vi "RemoveConnectionID.vi"(8 "ArrayIN":T1(array[cluster])=[{"IPaddress"="127.0.0.1", "Port"=63400, "connection ID"=refnum, "TCP error"={"status"=TRUE, "code"=1, "source"="TCP Write in TCPwrite8bytesMC.vi->PicoCmdClientMOVE-ForMasterControl_3.vi->Manual command_11.vi"}}], 11 "connection ID":refnum<k5>) -> (0 "ArrayOUT":T1(array[cluster])=[{"IPaddress"="127.0.0.1", "Port"=63400, "connection ID"=refnum, "TCP error"={"status"=TRUE, "code"=1, "source"="TCP Write in TCPwrite8bytesMC.vi->PicoCmdClientMOVE-ForMasterControl_3.vi->Manual command_11.vi"}}], 3 "Status":bool=TRUE)   [LabVIEW 2013]
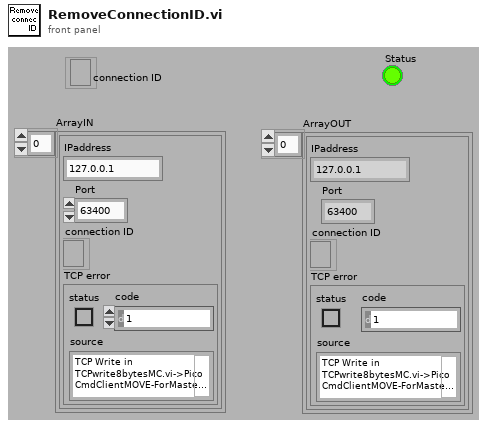
[diagram p1: front panel]
types:
  T1 = cluster{"IPaddress":string, "Port":i32, "connection ID":refnum<k5>, "TCP error":errorcluster}[]
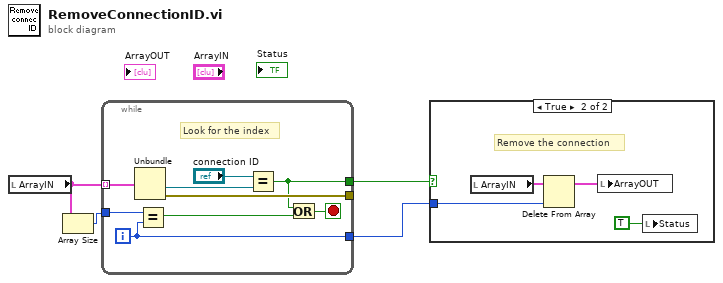
[diagram p0: block diagram]
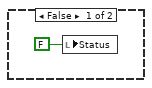
[diagram p2: hidden frame]
diagram:
  n1 = local read "ArrayIN"() -> (w4:T1)
  n2 = Array Size(array=w4) -> (size(s)=w3:i32)
  n3 = while {
    tunnel: w4 -> [w13] mode=indexing
    tunnel: w3 -> [w12]
    tunnel: [w11] -> _
    tunnel: [w7] -> w1
    tunnel: [w8] -> w2
    i -> [w8]
    stop <- w5 stop-if-true
    # "Look for the index"
    n4 = Unbundle(w13) -> ("connection ID"=w9:refnum<k5>, "TCP error"=w11:errorcluster)  [unwired: 2 out]
    n5 = Equal?(x=w12, y=w8) -> (x = y?=w6:bool)
    n6 = Equal?(x="connection ID", y=w9) -> (x = y?=w7:bool)
    n7 = Or(x=w7, y=w6) -> (x .or. y?=w5:bool)
  }
  n8 = case shown="True" w1 {
    tunnel: w2 -> [_ w15]
    frame False {
      n9 = local write "Status"(FALSE ("Status")) -> ()
    }
    frame True {
      # "Remove the connection"
      n10 = local read "ArrayIN"() -> (w18:T1)
      n11 = Delete From Array(array=w18, index=w15) -> (array with subset deleted=w17:T1)  [unwired: 1 in, 1 out]
      n12 = local write "ArrayOUT"(w17) -> ()
      n13 = local write "Status"(TRUE ("Status")) -> ()
    }
  }
